vi "INITIALISE XYZ STAGE CONTROLLER.vi"(8 "error in (no error)":errorcluster, 10 "INIITIALISE":string[](array[string])=["TOC=5000", "EO=15", "ABS", "IERR=0"], 11 "APERTURE IN":refnum<visa-resource-name>) -> (0 "ERROR OUT":errorcluster, 1 "VALID SESSION":bool, 2 "TCP/IP Settings:Dot-Notation Address":string, 3 "APERTURE OUT":refnum<visa-resource-name>, 4 "OUTPUT":string[](array[string]))   [LabVIEW 2018]
uses:
  <vilib>/Instr/_visa.llb/VISA Open Access Mode.ctl
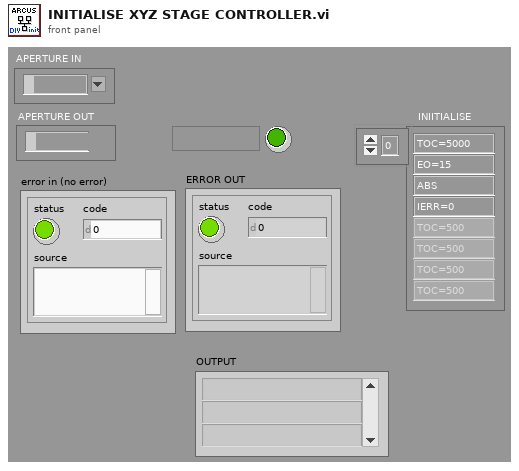
[diagram p1: front panel]
types:
  T1 = typedef "VISA Open Access Mode.ctl" = u32
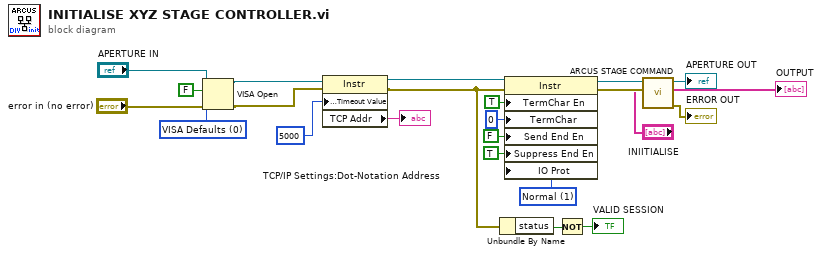
[diagram p0: block diagram]
diagram:
  w11 = u16 1 items=["Normal"=1, "VXI/FDC"=2, "GPIB/HS488"=3, "Serial-TCPIP-USB/488 Strings"=4, "USBTMC/Vendor-Specific"=5] ("Message Based Settings:IO Protocol")
  w23 = T1 0 items=["VISA Defaults"=0, "Exclusive Lock"=1, "Load Configured Settings"=4] ("Access Mode")
  n1 = VISA Open(duplicate session (F)=FALSE, access mode=w23, error in (no error)="error in (no error)", VISA resource name="APERTURE IN") -> (VISA resource name=w7:refnum<visa-resource-name>, error out=w6:errorcluster)  [unwired: 1 in]
  n2 = property class="Instr"(reference=w7, error in=w6, "General Settings:Timeout Value"=u32 5000) -> (reference out=w16:refnum<visa-resource-name>, error out=w15:errorcluster, "TCP Addr"=→"TCP/IP Settings:Dot-Notation Address":string)
  n3 = Unbundle By Name(w15) -> ("status"=w14:bool)
  n4 = property class="Instr"(reference=w16, error in=w15, "TermChar En"=TRUE ("Message Based Settings:Termination Character Enable"), "TermChar"=u8 0 ("Message Based Settings:Termination Character"), "Send End En"=FALSE ("Message Based Settings:Send End Enable"), "Suppress End En"=TRUE ("Message Based Settings:Suppress End Enable"), "IO Prot"=w11) -> (reference out=w20:refnum<visa-resource-name>, error out=w19:errorcluster)
  n5 = Not(x=w14) -> (.not. x?=→"VALID SESSION":bool)
  n6 = call "ARCUS STAGE COMMAND.vi"("error in (no error)"=w19, "COMMANDS"="INIITIALISE", "OBJECT IN"=w20) -> ("error out"=→"ERROR OUT":errorcluster, "OUTPUT"=→"OUTPUT":string[], "OBJECT OUT"=→"APERTURE OUT":refnum<visa-resource-name>)  [unwired: 6 in]
